vi "rsidr_core_global.vi"() -> ()   [LabVIEW 2020, in "Rohde&Schwarz RTx Oscilloscopes.lvlib"] (continued)
"Read Callback"="", "Write Callback"="", "Supported Models"="", "Instrument Options"="", "Flags"=0, "Help"="Defines the cursor measurement type.\n\nAvailable Repeated Capabilities:\nNone\n\nRemote-control command(s):\nCURSor<m>:FUNCtion"}, {"Level"=2, "Class Only"=FALSE, "Identifier"="RSRTX_ATTR_CURSOR_SOURCE", "Descriptive Name"="Cursor Source", "Data Type"=0, "Command"="CURS1:SOUR", "Access"=2, "Range Table"="rsrtx_rngWaveformParameter", "Read Callback"="", "Write Callback"="", "Supported Models"="", "Instrument Options"="", "Flags"=0, "Help"="Defines the source of the cursor measurement.\n\nAvailable Repeated Capabilities:\nNone\n\nRemote-control command(s):\nCURSor<m>:SOURce"}, {"Level"=2, "Class Only"=FALSE, "Identifier"="RSRTX_ATTR_CURSOR_SECOND_SOURCE", "Descriptive Name"="Cursor Second Source", "Data Type"=0, "Command"="CURS:SSO", "Access"=2, "Range Table"="rsrtx_rngWaveformParameter", "Read Callback"="", "Write Callback"="", "Supported Models"="", "Instrument Options"="", "Flags"=0, "Help"="Selects the second cursor source.\n\nAvailable Repeated Capabilities:\nNone\n\nRemote-control command(s):\nCURSor<m>:SSOURce"}, {"Level"=2, "Class Only"=FALSE, "Identifier"="RSRTX_ATTR_CURSOR_SECOND_SOURCE_ENABLE", "Descriptive Name"="Cursor Second Source Enable", "Data Type"=3, "Command"="CURS:USS", "Access"=2, "Range Table"="", "Read Callback"="", "Write Callback"="", "Supported Models"="", "Instrument Options"="", "Flags"=0, "Help"="Enables the second cursor source. To select the second source, use RSRTX_ATTR_CURSOR_SECOND_SOURCE. If enabled, the second cursor measures on the second source. Using a second source, you can measure differences between two waveforms with cursors. Both sources must be in the same domain (time domain or frequency domain).\n\nAvailable Repeated Capabilities:\nNone\n\nRemote-control command(s):\nCURSor<m>:USSOURce"}, {"Level"=2, "Class Only"=FALSE, "Identifier"="RSRTX_ATTR_CURSOR_TRACKING", "Descriptive Name"="Cursor Tracking", "Data Type"=3, "Command"="CURS1:TRAC", "Access"=2, "Range Table"="", "Read Callback"="", "Write Callback"="", "Supported Models"="", "Instrument Options"="", "Flags"=0, "Help"="If set to ON, the horizontal cursor lines follow the waveform.\n\nAvailable Repeated Capabilities:\nNone\n\nRemote-control command(s):\nCURSor<m>:TRACking[:STATe]"}, {"Level"=2, "Class Only"=FALSE, "Identifier"="RSRTX_ATTR_CURSOR_X_POSITION_COUPLING", "Descriptive Name"="Cursor X Position Coupling", "Data Type"=3, "Command"="CURS1:XCO", "Access"=2, "Range Table"="", "Read Callback"="", "Write Callback"="", "Supported Models"="", "Instrument Options"="", "Flags"=0, "Help"="Defines the positioning mode of the vertical cursor. \nON: Moving one cursor line moves the other cursor line too. The cursor lines always remain a fixed distance.\nOFF: Each cursor line is positioned independently.\n\nAvailable Repeated Capabilities:\nNone\n\nRemote-control command(s):\nCURSor<m>:XCOupling"}, {"Level"=2, "Class Only"=FALSE, "Identifier"="RSRTX_ATTR_CURSOR_Y_POSITION_COUPLING", "Descriptive Name"="Cursor Y Position Coupling", "Data Type"=3, "Command"="CURS:YCO", "Access"=2, "Range Table"="", "Read Callback"="", "Write Callback"="", "Supported Models"="", "Instrument Options"="", "Flags"=0, "Help"="Defines the positioning mode of the horizontal cursor. If the horizontal cursor lines track the waveform, the y-coupling is irrelevant.\nON: Moving one cursor line moves the other cursor line too. The cursor lines always remain a fixed distance.\nOFF: Each cursor line is positioned independently.\n\nAvailable Repeated Capabilities:\nNone\n\nRemote-control command(s):\nCURSor<m>:YCOupling"}, {"Level"=2, "Class Only"=FALSE, "Identifier"="RSRTX_ATTR_CURSOR_ADJUSTMENT", "Descriptive Name"="Cursor Adjustment", "Data Type"=3, "Command"="CURS1:TRAC:SCAL", "Access"=2, "Range Table"="", "Read Callback"="", "Write Callback"="", "Supported Models"="", "Instrument Options"="", "Flags"=0, "Help"="Enables the adjustment of cursor lines if the vertical or horizontal scales are changed.\n\nAvailable Repeated Capabilities:\nNone\n\nRemote-control command(s):\nCURSor<m>:TRACking:SCALe[:STATe]"}, {"Level"=2, "Class Only"=FALSE, "Identifier"="RSRTX_ATTR_CURSOR_X_RATIO_MEASUREMENT_UNIT", "Descriptive Name"="Cursor X Ratio Measurement Unit", "Data Type"=0, "Command"="CURS1:XRAT:UNIT", "Access"=2, "Range Table"="rsrtx_rngXRatioMeasurementUnit", "Read Callback"="", "Write Callback"="", "Supported Models"="", "Instrument Options"="", "Flags"=0, "Help"="Sets the unit for X Ratio measurements.\n\nAvailable Repeated Capabilities:\nNone\n\nRemote-control command(s):\nCURsor<m>:XRATio:UNIT"}, {"Level"=2, "Class Only"=FALSE, "Identifier"="RSRTX_ATTR_CURSOR_Y_RATIO_MEASUREMENT_UNIT", "Descriptive Name"="Cursor Y Ratio Measurement Unit", "Data Type"=0, "Command"="CURS1:YRAT:UNIT", "Access"=2, "Range Table"="rsrtx_rngYRatioMeasurementUnit", "Read Callback"="", "Write Callback"="", "Supported Models"="", "Instrument Options"="", "Flags"=0, "Help"="Sets the unit for Y Ratio measurements.\n\nAvailable Repeated Capabilities:\nNone\n\nRemote-control command(s):\nCURSor<m>:YRATio:UNIT"}, {"Level"=2, "Class Only"=FALSE, "Identifier"="RSRTX_ATTR_CURSOR_X_RATIO_MEASUREMENT", "Descriptive Name"="Cursor X Ratio Measurement", "Data Type"=1, "Command"="CURS1:XRAT?", "Access"=0, "Range Table"="", "Read Callback"="", "Write Callback"="", "Supported Models"="", "Instrument Options"="", "Flags"=0, "Help"="Returns the ratio of the x-values (e.g. a duty cycle) between the first and second cursors and the first and third cursors: (x2-x1)/(x3-x1).\n\nAvailable Repeated Capabilities:\nNone\n\nRemote-control command(s):\nCURSor<m>:XRATio[:VALue]?"}, {"Level"=2, "Class Only"=FALSE, "Identifier"="RSRTX_ATTR_CURSOR_Y_RATIO_MEASUREMENT", "Descriptive Name"="Cursor Y Ratio Measurement", "Data Type"=1, "Command"="CURS1:YRAT?", "Access"=0, "Range Table"="", "Read Callback"="", "Write Callback"="", "Supported Models"="", "Instrument Options"="", "Flags"=0, "Help"="Provides three cursors and measures the ratio of the y-values (e.g. overshooting) between the first and second cursors and the first and third cursors: (y2-y1)/(y3-y1).\n\nAvailable Repeated Capabilities:\nNone\n\nRemote-control command(s):\nCURSor<m>:YRATio[:VALue]?"}, {"Level"=2, "Class Only"=FALSE, "Identifier"="RSRTX_ATTR_CURSOR_DISTANCE_HORIZONTAL", "Descriptive Name"="Cursor Distance Horizontal", "Data Type"=1, "Command"="CURS1:XDEL?", "Access"=0, "Range Table"="", "Read Callback"="", "Write Callback"="", "Supported Models"="", "Instrument Options"="", "Flags"=0, "Help"="Queries the delta value (distance) of two horizontal cursors.\n\nAvailable Repeated Capabilities:\nNone\n\nRemote-control command(s):\nCURSor<m>:XDELta[:VALue]?"}, {"Level"=2, "Class Only"=FALSE, "Identifier"="RSRTX_ATTR_CURSOR_DISTANCE_VERTICAL", "Descriptive Name"="Cursor Distance Vertical", "Data Type"=1, "Command"="CURS1:YDEL?", "Access"=0, "Range Table"="", "Read Callback"="", "Write Callback"="", "Supported Models"="", "Instrument Options"="", "Flags"=0, "Help"="Queries the delta value (distance) of two vertical cursors.\n\nAvailable Repeated Capabilities:\nNone\n\nRemote-control command(s):\nCURSor<m>:YDELta[:VALue]?"}, {"Level"=2, "Class Only"=FALSE, "Identifier"="RSRTX_ATTR_CURSOR_INVERSE_DISTANCE", "Descriptive Name"="Cursor Inverse Distance", "Data Type"=1, "Command"="CURS1:XDEL:INV?", "Access"=0, "Range Table"="", "Read Callback"="", "Write Callback"="", "Supported Models"="", "Instrument Options"="", "Flags"=0, "Help"="Queries the inverse value of the delta value (distance) of the two vertical or horizontal cursors,\n\nAvailable Repeated Capabilities:\nNone\n\nRemote-control command(s):\nCURSor<m>:XDELta:INVerse?"}, {"Level"=2, "Class Only"=FALSE, "Identifier"="RSRTX_ATTR_CURSOR_VOLTAGE_INVERSE_DISTANCE_VERTICAL", "Descriptive Name"="Cursor Voltage Inverse Distance Vertical", "Data Type"=1, "Command"="CURS1:YDEL:SLOP?", "Access"=0, "Range Table"="", "Read Callback"="", "Write Callback"="", "Supported Models"="", "Instrument Options"="", "Flags"=1, "Help"="Returns the inverse value of the voltage difference - the reciprocal of the vertical distance of two horizontal cursor lines: 1/?V.\n\nAvailable Repeated Capabilities:\nNone\n\nRemote-control command(s):\nCURSor<m>:YDELta:SLOPe?"}, {"Level"=2, "Class Only"=FALSE, "Identifier"="RSRTX_ATTR_CURSOR_POSITION", "Descriptive Name"="Cursor Position", "Data Type"=1, "Command"="CURS1:RESult?", "Access"=0, "Range Table"="", "Read Callback"="", "Write Callback"="", "Supported Models"="", "Instrument Options"="", "Flags"=1, "Help"="Returns the cursor positions.\n\nAvailable Repeated Capabilities:\nNone\n\nRemote-control command(s):\nCURSor<m>:RESult?"}, {"Level"=2, "Class Only"=FALSE, "Identifier"="RSRTX_ATTR_CURSOR_AUTOSET", "Descriptive Name"="Cursor Autoset", "Data Type"=4, "Command"="CURS{Cursor}:SWAV", "Access"=1, "Range Table"="", "Read Callback"="", "Write Callback"="", "Supported Models"="", "Instrument Options"="", "Flags"=1, "Help"="Sets the cursor lines to typical points of the waveform depending on the selected measurement type.\n\nAvailable Repeated Capabilities:\nCursor: Cur1, Cur2, Cur3\r\n\nRemote-control command(s):\nCURSor<m>:SWAVe"}, {"Level"=2, "Class Only"=FALSE, "Identifier"="RSRTX_ATTR_CURSOR_RESET", "Descriptive Name"="Cursor Reset", "Data Type"=4, "Command"="CURS{Cursor}:SSCR", "Access"=1, "Range Table"="", "Read Callback"="", "Write Callback"="", "Supported Models"="", "Instrument Options"="", "Flags"=0, "Help"="Resets the cursors to their initial positions.\n\nAvailable Repeated Capabilities:\nCursor: Cur1, Cur2, Cur3\r\n\nRemote-control command(s):\nCURSor<m>:SSCReen"}, {"Level"=2, "Class Only"=FALSE, "Identifier"="RSRTX_ATTR_CURSOR_PEAK_NEXT", "Descriptive Name"="Cursor Peak Next", "Data Type"=4, "Command"="CURS{Cursor}:SNP", "Access"=1, "Range Table"="", "Read Callback"="", "Write Callback"="", "Supported Models"="", "Instrument Options"="", "Flags"=0, "Help"="Sets cursor to the next peak.\n\nAvailable Repeated Capabilities:\nCursor: Cur1, Cur2, Cur3\r\n\nRemote-control command(s):\nCURSor<m>:SNPeak"}, {"Level"=2, "Class Only"=FALSE, "Identifier"="RSRTX_ATTR_CURSOR_PEAK_PREVIOUS", "Descriptive Name"="Cursor Peak Previous", "Data Type"=4, "Command"="CURS{Cursor}:SPP", "Access"=1, "Range Table"="", "Read Callback"="", "Write Callback"="", "Supported Models"="", "Instrument Options"="", "Flags"=0, "Help"="Sets cursor to the previous peak.\n\nAvailable Repeated Capabilities:\nCursor: Cur1, Cur2, Cur3\r\n\nRemote-control command(s):\nCURSor<m>:SPPeak"}, {"Level"=2, "Class Only"=FALSE, "Identifier"="RSRTX_ATTR_CURSOR_X1_POSITION", "Descriptive Name"="Cursor X1 Position", "Data Type"=1, "Command"="CURS1:X1P", "Access"=2, "Range Table"="rsrtx_rngCursorXPosition", "Read Callback"="", "Write Callback"="", "Supported Models"="", "Instrument Options"="", "Flags"=0, "Help"="Defines the vertical position of first cursor or cursor line.\n\nAvailable Repeated Capabilities:\nNone\n\nRemote-control command(s):\nCURSor<m>:X1Position"}, {"Level"=2, "Class Only"=FALSE, "Identifier"="RSRTX_ATTR_CURSOR_X2_POSITION", "Descriptive Name"="Cursor X2 Position", "Data Type"=1, "Command"="CURS1:X2P", "Access"=2, "Range Table"="rsrtx_rngCursorXPosition", "Read Callback"="", "Write Callback"="", "Supported Models"="", "Instrument Options"="", "Flags"=0, "Help"="Defines the vertical position of second cursor or cursor line.\n\nAvailable Repeated Capabilities:\nNone\n\nRemote-control command(s):\nCURSor<m>:X2Position"}, {"Level"=2, "Class Only"=FALSE, "Identifier"="RSRTX_ATTR_CURSOR_X3_POSITION", "Descriptive Name"="Cursor X3 Position", "Data Type"=1, "Command"="CURS1:X3P", "Access"=2, "Range Table"="rsrtx_rngCursorXPosition", "Read Callback"="", "Write Callback"="", "Supported Models"="", "Instrument Options"="", "Flags"=0, "Help"="Defines the vertical position of third cursor or cursor line.\n\nAvailable Repeated Capabilities:\nNone\n\nRemote-control command(s):\nCURSor<m>:X3Position"}, {"Level"=2, "Class Only"=FALSE, "Identifier"="RSRTX_ATTR_CURSOR_Y1_POSITION", "Descriptive Name"="Cursor Y1 Position", "Data Type"=1, "Command"="CURS1:Y1P", "Access"=2, "Range Table"="rsrtx_rngCursorYPosition", "Read Callback"="", "Write Callback"="", "Supported Models"="", "Instrument Options"="", "Flags"=0, "Help"="Defines the horizontal position of first cursor or cursor line.\n\nAvailable Repeated Capabilities:\nNone\n\nRemote-control command(s):\nCURSor<m>:Y1Position"}, {"Level"=2, "Class Only"=FALSE, "Identifier"="RSRTX_ATTR_CURSOR_Y2_POSITION", "Descriptive Name"="Cursor Y2 Position", "Data Type"=1, "Command"="CURS1:Y2P", "Access"=2, "Range Table"="rsrtx_rngCursorYPosition", "Read Callback"="", "Write Callback"="", "Supported Models"="", "Instrument Options"="", "Flags"=0, "Help"="Defines the horizontal position of second cursor or cursor line.\n\nAvailable Repeated Capabilities:\nNone\n\nRemote-control command(s):\nCURSor<m>:Y2Position"}, {"Level"=2, "Class Only"=FALSE, "Identifier"="RSRTX_ATTR_CURSOR_Y3_POSITION", "Descriptive Name"="Cursor Y3 Position", "Data Type"=1, "Command"="CURS1:Y3P", "Access"=2, "Range Table"="rsrtx_rngCursorYPosition", "Read Callback"="", "Write Callback"="", "Supported Models"="", "Instrument Options"="", "Flags"=0, "Help"="Defines the horizontal position of third cursor or cursor line.\n\nAvailable Repeated Capabilities:\nNone\n\nRemote-control command(s):\nCURSor<m>:Y3Position"}, {"Level"=2, "Class Only"=TRUE, "Identifier"="", "Descriptive Name"="Cursor Line", "Data Type"=0, "Command"="", "Access"=0, "Range Table"="", "Read Callback"="", "Write Callback"="", "Supported Models"="", "Instrument Options"="", "Flags"=0, "Help"="Class for CursorLine repcap."}, {"Level"=3, "Class Only"=FALSE, "Identifier"="RSRTX_ATTR_CURSOR_LINE_NEXT_PEAK", "Descriptive Name"="Cursor Line Next Peak", "Data Type"=4, "Command"="CURS{Cursor}:SNP{CursorLine}", "Access"=1, "Range Table"="", "Read Callback"="", "Write Callback"="", "Supported Models"="", "Instrument Options"="", "Flags"=0, "Help"="Set the cursor line to the next peak, respectively. Only available for FFT waveforms.\n\nAvailable Repeated Capabilities:\nCursor: Cur1, Cur2, Cur3\r\nCursorLine: CursorLine1, CursorLine2\r\n\nRemote-control command(s):\nCURSor<m>:SNPeak<n>"}, {"Level"=3, "Class Only"=FALSE, "Identifier"="RSRTX_ATTR_CURSOR_LINE_PREVIOUS_PEAK", "Descriptive Name"="Cursor Line Previous Peak", "Data Type"=4, "Command"="CURS{Cursor}:SPP{CursorLine}", "Access"=1, "Range Table"="", "Read Callback"="", "Write Callback"="", "Supported Models"="", "Instrument Options"="", "Flags"=0, "Help"="Set the cursor line to the previous peak, respectively. Only available for FFT waveforms.\n\nAvailable Repeated Capabilities:\nCursor: Cur1, Cur2, Cur3\r\nCursorLine: CursorLine1, CursorLine2\r\n\nRemote-control command(s):\nCURSor<m>:SPPeak<n>"}, {"Level"=1, "Class Only"=TRUE, "Identifier"="", "Descriptive Name"="Measurements", "Data Type"=0, "Command"="", "Access"=0, "Range Table"="", "Read Callback"="", "Write Callback"="", "Supported Models"="", "Instrument Options"="", "Flags"=0, "Help"="Configures scope measurements and queries results."}, {"Level"=2, "Class Only"=FALSE, "Identifier"="RSRTX_ATTR_MEAS_RELATIVE_MODE", "Descriptive Name"="Measurement Relative Mode", "Data Type"=0, "Command"="REFL:REL:MODE", "Access"=2, "Range Table"="rsrtx_rngRelativeMode", "Read Callback"="", "Write Callback"="", "Supported Models"="", "Instrument Options"="", "Flags"=0, "Help"="Sets the lower and upper reference levels for rise and fall time mesurements (cursor and automatic mesurements) as well as the middle reference level for phase and delay measurements. The levels are defined as percentages of the high signal level. The setting is valid for all measurement places.\n\nAvailable Repeated Capabilities:\nNone\n\nRemote-control command(s):\nREFLevel:RELative:MODE"}, {"Level"=2, "Class Only"=FALSE, "Identifier"="RSRTX_ATTR_MEAS_RELATIVE_LOWER_LEVEL", "Descriptive Name"="Measurement Relative Lower Level", "Data Type"=1, "Command"="REFL:REL:LOW", "Access"=2, "Range Table"="rsrtx_rngRelLevel", "Read Callback"="", "Write Callback"="", "Supported Models"="", "Instrument Options"="", "Flags"=0, "Help"="Set the lower reference level for rise and fall time mesurements.\n\nAvailable Repeated Capabilities:\nNone\n\nRemote-control command(s):\nREFLevel:RELative:LOWer"}, {"Level"=2, "Class Only"=FALSE, "Identifier"="RSRTX_ATTR_MEAS_RELATIVE_UPPER_LEVEL", "Descriptive Name"="Measurement Relative Upper Level", "Data Type"=1, "Command"="REFL:REL:UPP", "Access"=2, "Range Table"="rsrtx_rngRelLevel", "Read Callback"="", "Write Callback"="", "Supported Models"="", "Instrument Options"="", "Flags"=0, "Help"="Set the upper reference level for rise and fall time mesurements.\n\nAvailable Repeated Capabilities:\nNone\n\nRemote-control command(s):\nREFLevel:RELative:UPPer"}, {"Level"=2, "Class Only"=FALSE, "Identifier"="RSRTX_ATTR_MEAS_RELATIVE_MIDDLE_LEVEL", "Descriptive Name"="Measurement Relative Middle Level", "Data Type"=1, "Command"="REFL:REL:MIDD", "Access"=2, "Range Table"="rsrtx_rngRelLevel", "Read Callback"="", "Write Callback"="", "Supported Models"="", "Instrument Options"="", "Flags"=0, "Help"="Set the middle reference level used for phase and delay measurements.\n\nAvailable Repeated Capabilities:\nNone\n\nRemote-control command(s):\nREFLevel:RELative:MIDDle"}, {"Level"=2, "Class Only"=TRUE, "Identifier"="", "Descriptive Name"="Main Measurements", "Data Type"=0, "Command"="", "Access"=0, "Range Table"="", "Read Callback"="", "Write Callback"="", "Supported Models"="", "Instrument Options"="", "Flags"=0, "Help"="Configures scope measurements and queries results."}, {"Level"=3, "Class Only"=FALSE, "Identifier"="RSRTX_ATTR_MAIN_MEASUREMENT_RESULT_FREQUENCY", "Descriptive Name"="Main Measurement Result Frequency", "Data Type"=1, "Command"="MEAS{Measurement}:RES? FREQ", "Access"=0, "Range Table"="", "Read Callback"="", "Write Callback"="", "Supported Models"="", "Instrument Options"="", "Flags"=0, "Help"="Returns the result of the frequency measurement type.\n\nAvailable Repeated Capabilities:\nMeasurement: M1, M2, M3, M4, M5, M6, M7, M8\r\n\nRemote-control command(s):\nMEASurement<m>:RESult[:ACTual]?"}, {"Level"=3, "Class Only"=FALSE, "Identifier"="RSRTX_ATTR_MAIN_MEASUREMENT_RESULT_PERIOD", "Descriptive Name"="Main Measurement Result Period", "Data Type"=1, "Command"="MEAS{Measurement}:RES? PER", "Access"=0, "Range Table"="", "Read Callback"="", "Write Callback"="", "Supported Models"="", "Instrument Options"="", "Flags"=0, "Help"="Returns the result of the period measurement type.\n\nAvailable Repeated Capabilities:\nMeasurement: M1, M2, M3, M4, M5, M6, M7, M8\r\n\nRemote-control command(s):\nMEASurement<m>:RESult[:ACTual]?"}, {"Level"=3, "Class Only"=FALSE, "Identifier"="RSRTX_ATTR_MAIN_MEASUREMENT_RESULT_PEAK", "Descriptive Name"="Main Measurement Result Peak", "Data Type"=1, "Command"="MEAS{Measurement}:RES? PEAK", "Access"=0, "Range Table"="", "Read Callback"="", "Write Callback"="", "Supported Models"="", "Instrument Options"="", "Flags"=0, "Help"="Returns the result of the peak measurement type.\n\nAvailable Repeated Capabilities:\nMeasurement: M1, M2, M3, M4, M5, M6, M7, M8\r\n\nRemote-control command(s):\nMEASurement<m>:RESult[:ACTual]?"}, {"Level"=3, "Class Only"=FALSE, "Identifier"="RSRTX_ATTR_MAIN_MEASUREMENT_RESULT_MAXIMUM_PEAK", "Descriptive Name"="Main Measurement Result Maximum Peak", "Data Type"=1, "Command"="MEAS{Measurement}:RES? UPE", "Access"=0, "Range Table"="", "Read Callback"="", "Write Callback"="", "Supported Models"="", "Instrument Options"="", "Flags"=0, "Help"="Returns the result of the maximum peak measurement type.\n\nAvailable Repeated Capabilities:\nMeasurement: M1, M2, M3, M4, M5, M6, M7, M8\r\n\nRemote-control command(s):\nMEASurement<m>:RESult[:ACTual]?"}, {"Level"=3, "Class Only"=FALSE, "Identifier"="RSRTX_ATTR_MAIN_MEASUREMENT_RESULT_MINIMUM_PEAK", "Descriptive Name"="Main Measurement Result Minimum Peak", "Data Type"=1, "Command"="MEAS{Measurement}:RES? LPE", "Access"=0, "Range Table"="", "Read Callback"="", "Write Callback"="", "Supported Models"="", "Instrument Options"="", "Flags"=0, "Help"="Returns the result of the minimum peak measurement type.\n\nAvailable Repeated Capabilities:\nMeasurement: M1, M2, M3, M4, M5, M6, M7, M8\r\n\nRemote-control command(s):\nMEASurement<m>:RESult[:ACTual]?"}, {"Level"=3, "Class Only"=FALSE, "Identifier"="RSRTX_ATTR_MAIN_MEASUREMENT_RESULT_POSITIVE_PULSES", "Descriptive Name"="Main Measurement Result Positive Pulses", "Data Type"=1, "Command"="MEAS{Measurement}:RES? PPC", "Access"=0, "Range Table"="", "Read Callback"="", "Write Callback"="", "Supported Models"="", "Instrument Options"="", "Flags"=0, "Help"="Returns the result of the positive pulses measurement type.\n\nAvailable Repeated Capabilities:\nMeasurement: M1, M2, M3, M4, M5, M6, M7, M8\r\n\nRemote-control command(s):\nMEASurement<m>:RESult[:ACTual]?"}, {"Level"=3, "Class Only"=FALSE, "Identifier"="RSRTX_ATTR_MAIN_MEASUREMENT_RESULT_NEGATIVE_PULSES", "Descriptive Name"="Main Measurement Result Negative Pulses", "Data Type"=1, "Command"="MEAS{Measurement}:RES? NPC", "Access"=0, "Range Table"="", "Read Callback"="", "Write Callback"="", "Supported Models"="", "Instrument Options"="", "Flags"=0, "Help"="Returns the result of the negative pulses measurement type.\n\nAvailable Repeated Capabilities:\nMeasurement: M1, M2, M3, M4, M5, M6, M7, M8\r\n\nRemote-control command(s):\nMEASurement<m>:RESult[:ACTual]?"}, {"Level"=3, "Class Only"=FALSE, "Identifier"="RSRTX_ATTR_MAIN_MEASUREMENT_RESULT_RISING_EDGES", "Descriptive Name"="Main Measurement Result Rising Edges", "Data Type"=1, "Command"="MEAS{Measurement}:RES? REC", "Access"=0, "Range Table"="", "Read Callback"="", "Write Callback"="", "Supported Models"="", "Instrument Options"="", "Flags"=0, "Help"="Returns the result of the rising edges measurement type.\n\nAvailable Repeated Capabilities:\nMeasurement: M1, M2, M3, M4, M5, M6, M7, M8\r\n\nRemote-control command(s):\nMEASurement<m>:RESult[:ACTual]?"}, {"Level"=3, "Class Only"=FALSE, "Identifier"="RSRTX_ATTR_MAIN_MEASUREMENT_RESULT_FALLING_EDGES", "Descriptive Name"="Main Measurement Result Falling Edges", "Data Type"=1, "Command"="MEAS{Measurement}:RES? FEC", "Access"=0, "Range Table"="", "Read Callback"="", "Write Callback"="", "Supported Models"="", "Instrument Options"="", "Flags"=0, "Help"="Returns the result of the falling edges measurement type.\n\nAvailable Repeated Capabilities:\nMeasurement: M1, M2, M3, M4, M5, M6, M7, M8\r\n\nRemote-control command(s):\nMEASurement<m>:RESult[:ACTual]?"}, {"Level"=3, "Class Only"=FALSE, "Identifier"="RSRTX_ATTR_MAIN_MEASUREMENT_RESULT_HIGH_LEVEL", "Descriptive Name"="Main Measurement Result High Level", "Data Type"=1, "Command"="MEAS{Measurement}:RES? HIGH", "Access"=0, "Range Table"="", "Read Callback"="", "Write Callback"="", "Supported Models"="", "Instrument Options"="", "Flags"=0, "Help"="Returns the result of the high level measurement type.\n\nAvailable Repeated Capabilities:\nMeasurement: M1, M2, M3, M4, M5, M6, M7, M8\r\n\nRemote-control command(s):\nMEASurement<m>:RESult[:ACTual]?"}, {"Level"=3, "Class Only"=FALSE, "Identifier"="RSRTX_ATTR_MAIN_MEASUREMENT_RESULT_LOW_LEVEL", "Descriptive Name"="Main Measurement Result Low Level", "Data Type"=1, "Command"="MEAS{Measurement}:RES? LOW", "Access"=0, "Range Table"="", "Read Callback"="", "Write Callback"="", "Supported Models"="", "Instrument Options"="", "Flags"=0, "Help"="Returns the result of the low level measurement type.\n\nAvailable Repeated Capabilities:\nMeasurement: M1, M2, M3, M4, M5, M6, M7, M8\r\n\nRemote-control command(s):\nMEASurement<m>:RESult[:ACTual]?"}, {"Level"=3, "Class Only"=FALSE, "Identifier"="RSRTX_ATTR_MAIN_MEASUREMENT_RESULT_AMPLITUDE", "Descriptive Name"="Main Measurement Result Amplitude", "Data Type"=1, "Command"="MEAS{Measurement}:RES? AMPL", "Access"=0, "Range Table"="", "Read Callback"="", "Write Callback"="", "Supported Models"="", "Instrument Options"="", "Flags"=0, "Help"="Returns the result of the amplitude measurement type.\n\nAvailable Repeated Capabilities:\nMeasurement: M1, M2, M3, M4, M5, M6, M7, M8\r\n\nRemote-control command(s):\nMEASurement<m>:RESult[:ACTual]?"}, {"Level"=3, "Class Only"=FALSE, "Identifier"="RSRTX_ATTR_MAIN_MEASUREMENT_RESULT_MEAN", "Descriptive Name"="Main Measurement Result Mean", "Data Type"=1, "Command"="MEAS{Measurement}:RES? MEAN", "Access"=0, "Range Table"="", "Read Callback"="", "Write Callback"="", "Supported Models"="", "Instrument Options"="", "Flags"=0, "Help"="Returns the result of the mean measurement type.\n\nAvailable Repeated Capabilities:\nMeasurement: M1, M2, M3, M4, M5, M6, M7, M8\r\n\nRemote-control command(s):\nMEASurement<m>:RESult[:ACTual]?"}, {"Level"=3, "Class Only"=FALSE, "Identifier"="RSRTX_ATTR_MAIN_MEASUREMENT_RESULT_RMS", "Descriptive Name"="Main Measurement Result RMS", "Data Type"=1, "Command"="MEAS{Measurement}:RES? RMS", "Access"=0, "Range Table"="", "Read Callback"="", "Write Callback"="", "Supported Models"="", "Instrument Options"="", "Flags"=0, "Help"="Returns the result of the RMS measurement type.\n\nAvailable Repeated Capabilities:\nMeasurement: M1, M2, M3, M4, M5, M6, M7, M8\r\n\nRemote-control command(s):\nMEASurement<m>:RESult[:ACTual]?"}, {"Level"=3, "Class Only"=FALSE, "Identifier"="RSRTX_ATTR_MAIN_MEASUREMENT_RESULT_RISE_TIME", "Descriptive Name"="Main Measurement Result Rise Time", "Data Type"=1, "Command"="MEAS{Measurement}:RES? RTIM", "Access"=0, "Range Table"="", "Read Callback"="", "Write Callback"="", "Supported Models"="", "Instrument Options"="", "Flags"=0, "Help"="Returns the result of the rise time measurement type.\n\nAvailable Repeated Capabilities:\nMeasurement: M1, M2, M3, M4, M5, M6, M7, M8\r\n\nRemote-control command(s):\nMEASurement<m>:RESult[:ACTual]?"}, {"Level"=3, "Class Only"=FALSE, "Identifier"="RSRTX_ATTR_MAIN_MEASUREMENT_RESULT_FALLING_TIME", "Descriptive Name"="Main Measurement Result Falling Time", "Data Type"=1, "Command"="MEAS{Measurement}:RES? FTIM", "Access"=0, "Range Table"="", "Read Callback"="", "Write Callback"="", "Supported Models"="", "Instrument Options"="", "Flags"=0, "Help"="Returns the result of the falling time measurement type.\n\nAvailable Repeated Capabilities:\nMeasurement: M1, M2, M3, M4, M5, M6, M7, M8\r\n\nRemote-control command(s):\nMEASurement<m>:RESult[:ACTual]?"}, {"Level"=3, "Class Only"=FALSE, "Identifier"="RSRTX_ATTR_MAIN_MEASUREMENT_RESULT_POSITIVE_CYCLE", "Descriptive Name"="Main Measurement Result Positive Cycle", "Data Type"=1, "Command"="MEAS{Measurement}:RES? PDCY", "Access"=0, "Range Table"="", "Read Callback"="", "Write Callback"="", "Supported Models"="", "Instrument Options"="", "Flags"=0, "Help"="Returns the result of the positive cycle measurement type.\n\nAvailable Repeated Capabilities:\nMeasurement: M1, M2, M3, M4, M5, M6, M7, M8\r\n\nRemote-control command(s):\nMEASurement<m>:RESult[:ACTual]?"}, {"Level"=3, "Class Only"=FALSE, "Identifier"="RSRTX_ATTR_MAIN_MEASUREMENT_RESULT_NEGATIVE_CYCLE", "Descriptive Name"="Main Measurement Result Negative Cycle", "Data Type"=1, "Command"="MEAS{Measurement}:RES? NDCY", "Access"=0, "Range Table"="", "Read Callback"="", "Write Callback"="", "Supported Models"="", "Instrument Options"="", "Flags"=0, "Help"="Returns the result of the negative cycle measurement type.\n\nAvailable Repeated Capabilities:\nMeasurement: M1, M2, M3, M4, M5, M6, M7, M8\r\n\nRemote-control command(s):\nMEASurement<m>:RESult[:ACTual]?"}, {"Level"=3, "Class Only"=FALSE, "Identifier"="RSRTX_ATTR_MAIN_MEASUREMENT_RESULT_WIDTH_POSITIVE_PULSE", "Descriptive Name"="Main Measurement Result Width Positive Pulse", "Data Type"=1, "Command"="MEAS{Measurement}:RES? PPW", "Access"=0, "Range Table"="", "Read Callback"="", "Write Callback"="", "Supported Models"="", "Instrument Options"="", "Flags"=0, "Help"="Returns the result of the width of the positive pulse measurement type.\n\nAvailable Repeated Capabilities:\nMeasurement: M1, M2, M3, M4, M5, M6, M7, M8\r\n\nRemote-control command(s):\nMEASurement<m>:RESult[:ACTual]?"}, {"Level"=3, "Class Only"=FALSE, "Identifier"="RSRTX_ATTR_MAIN_MEASUREMENT_RESULT_WIDTH_NEGATIVE_PULSE", "Descriptive Name"="Main Measurement Result Width Negative Pulse", "Data Type"=1, "Command"="MEAS{Measurement}:RES? NPW", "Access"=0, "Range Table"="", "Read Callback"="", "Write Callback"="", "Supported Models"="", "Instrument Options"="", "Flags"=0, "Help"="Returns the result of the width of the negative pulse measurement type.\n\nAvailable Repeated Capabilities:\nMeasurement: M1, M2, M3, M4, M5, M6, M7, M8\r\n\nRemote-control command(s):\nMEASurement<m>:RESult[:ACTual]?"}, {"Level"=3, "Class Only"=FALSE, "Identifier"="RSRTX_ATTR_MAIN_MEASUREMENT_RESULT_MEAN_VALUE", "Descriptive Name"="Main Measurement Result Mean Value", "Data Type"=1, "Command"="MEAS{Measurement}:RES? CYCM", "Access"=0, "Range Table"="", "Read Callback"="", "Write Callback"="", "Supported Models"="", "Instrument Options"="", "Flags"=0, "Help"="Returns the result of the width of the mean value measurement type.\n\nAvailable Repeated Capabilities:\nMeasurement: M1, M2, M3, M4, M5, M6, M7, M8\r\n\nRemote-control command(s):\nMEASurement<m>:RESult[:ACTual]?"}, {"Level"=3, "Class Only"=FALSE, "Identifier"="RSRTX_ATTR_MAIN_MEASUREMENT_RESULT_RMS_VALUE", "Descriptive Name"="Main Measurement Result RMS Value", "Data Type"=1, "Command"="MEAS{Measurement}:RES? CYCR", "Access"=0, "Range Table"="", "Read Callback"="", "Write Callback"="", "Supported Models"="", "Instrument Options"="", "Flags"=0, "Help"="Returns the result of the width of the RMS value measurement type.\n\nAvailable Repeated Capabilities:\nMeasurement: M1, M2, M3, M4, M5, M6, M7, M8\r\n\nRemote-control command(s):\nMEASurement<m>:RESult[:ACTual]?"}, {"Level"=3, "Class Only"=FALSE, "Identifier"="RSRTX_ATTR_MAIN_MEASUREMENT_RESULT_STANDARD_DEVIATIONS", "Descriptive Name"="Main Measurement Result Standard Deviations", "Data Type"=1, "Command"="MEAS{Measurement}:RES? STDD", "Access"=0, "Range Table"="", "Read Callback"="", "Write Callback"="", "Supported Models"="", "Instrument Options"="", "Flags"=0, "Help"="Returns the result of the width of the standard deviation measurement type.\n\nAvailable Repeated Capabilities:\nMeasurement: M1, M2, M3, M4, M5, M6, M7, M8\r\n\nRemote-control command(s):\nMEASurement<m>:RESult[:ACTual]?"}, {"Level"=3, "Class Only"=FALSE, "Identifier"="RSRTX_ATTR_MAIN_MEASUREMENT_RESULT_STANDARD_DEVIATION_VALUE", "Descriptive Name"="Main Measurement Result Standard Deviation Value", "Data Type"=1, "Command"="MEAS{Measurement}:RES? CYCS", "Access"=0, "Range Table"="", "Read Callback"="", "Write Callback"="", "Supported Models"="", "Instrument Options"="", "Flags"=0, "Help"="Returns the result of the width of the standard deviation value measurement type.\n\nAvailable Repeated Capabilities:\nMeasurement: M1, M2, M3, M4, M5, M6, M7, M8\r\n\nRemote-control command(s):\nMEASurement<m>:RESult[:ACTual]?"}, {"Level"=3, "Class Only"=FALSE, "Identifier"="RSRTX_ATTR_MAIN_MEASUREMENT_RESULT_DELAY", "Descriptive Name"="Main Measurement Result Delay", "Data Type"=1, "Command"="MEAS{Measurement}:RES? DEL", "Access"=0, "Range Table"="", "Read Callback"="", "Write Callback"="", "Supported Models"="", "Instrument Options"="", "Flags"=0, "Help"="Returns the result of the width of the delay measurement type.\n\nAvailable Repeated Capabilities:\nMeasurement: M1, M2, M3, M4, M5, M6, M7, M8\r\n\nRemote-control command(s):\nMEASurement<m>:RESult[:ACTual]?"}, {"Level"=3, "Class Only"=FALSE, "Identifier"="RSRTX_ATTR_MAIN_MEASUREMENT_RESULT_PHASE", "Descriptive Name"="Main Measurement Result Phase", "Data Type"=1, "Command"="MEAS{Measurement}:RES? PHAS", "Access"=0, "Range Table"="", "Read Callback"="", "Write Callback"="", "Supported Models"="", "Instrument Options"="", "Flags"=0, "Help"="Returns the result of the width of the phase measurement type.\n\nAvailable Repeated Capabilities:\nMeasurement: M1, M2, M3, M4, M5, M6, M7, M8\r\n\nRemote-control command(s):\nMEASurement<m>:RESult[:ACTual]?"}, {"Level"=3, "Class Only"=FALSE, "Identifier"="RSRTX_ATTR_MAIN_MEASUREMENT_RESULT_BURST_WIDTH", "Descriptive Name"="Main Measurement Result Burst Width", "Data Type"=1, "Command"="MEAS{Measurement}:RES? BWID", "Access"=0, "Range Table"="", "Read Callback"="", "Write Callback"="", "Supported Models"="", "Instrument Options"="", "Flags"=0, "Help"="Returns the result of the width of the burst width measurement type.\n\nAvailable Repeated Capabilities:\nMeasurement: M1, M2, M3, M4, M5, M6, M7, M8\r\n\nRemote-control command(s):\nMEASurement<m>:RESult[:ACTual]?"}, {"Level"=3, "Class Only"=FALSE, "Identifier"="RSRTX_ATTR_MAIN_MEASUREMENT_RESULT_POSITIVE_OVERSHOOT", "Descriptive Name"="Main Measurement Result Positive Overshoot", "Data Type"=1, "Command"="MEAS{Measurement}:RES? POV", "Access"=0, "Range Table"="", "Read Callback"="", "Write Callback"="", "Supported Models"="", "Instrument Options"="", "Flags"=0, "Help"="Returns the result of the width of the positive overshoot measurement type.\n\nAvailable Repeated Capabilities:\nMeasurement: M1, M2, M3, M4, M5, M6, M7, M8\r\n\nRemote-control command(s):\nMEASurement<m>:RESult[:ACTual]?"}, {"Level"=3, "Class Only"=FALSE, "Identifier"="RSRTX_ATTR_MAIN_MEASUREMENT_RESULT_NEGATIVE_OVERSHOOT", "Descriptive Name"="Main Measurement Result Negative Overshoot", "Data Type"=1, "Command"="MEAS{Measurement}:RES? NOV", "Access"=0, "Range Table"="", "Read Callback"="", "Write Callback"="", "Supported Models"="", "Instrument Options"="", "Flags"=0, "Help"="Returns the result of the width of the negative overshoot measurement type.\n\nAvailable Repeated Capabilities:\nMeasurement: M1, M2, M3, M4, M5, M6, M7, M8\r\n\nRemote-control command(s):\nMEASurement<m>:RESult[:ACTual]?"}, {"Level"=3, "Class Only"=FALSE, "Identifier"="RSRTX_ATTR_MAIN_MEASUREMENT_RESULT_AVERAGE_VALUE", "Descriptive Name"="Main Measurement Result Average Value", "Data Type"=1, "Command"="MEAS{Measurement}:RES:AVG?", "Access"=0, "Range Table"="", "Read Callback"="", "Write Callback"="", "Supported Models"="", "Instrument Options"="", "Flags"=0, "Help"="Returns the result of the Average Value measurement type.\n\nAvailable Repeated Capabilities:\nMeasurement: M1, M2, M3, M4, M5, M6, M7, M8\r\n\nRemote-control command(s):\nMEASurement<m>:RESult:AVG?"}, {"Level"=3, "Class Only"=FALSE, "Identifier"="RSRTX_ATTR_MAIN_MEASUREMENT_RESULT_STANDARD_DEVIATION", "Descriptive Name"="Main Measurement Result Standard Deviation", "Data Type"=1, "Command"="MEAS{Measurement}:RES:STDD?", "Access"=0, "Range Table"="", "Read Callback"="", "Write Callback"="", "Supported Models"="", "Instrument Options"="", "Flags"=0, "Help"="Returns the result of the Standard Deviation measurement type.\n\nAvailable Repeated Capabilities:\nMeasurement: M1, M2, M3, M4, M5, M6, M7, M8\r\n\nRemote-control command(s):\nMEASurement<m>:RESult:STDDev?"}, {"Level"=3, "Class Only"=FALSE, "Identifier"="RSRTX_ATTR_MAIN_MEASUREMENT_RESULT_NEGATIVE_PEAK", "Descriptive Name"="Main Measurement Result Negative Peak", "Data Type"=1, "Command"="MEAS{Measurement}:RES:NPE?", "Access"=0, "Range Table"="", "Read Callback"="", "Write Callback"="", "Supported Models"="", "Instrument Options"="", "Flags"=0, "Help"="Returns the result of the Negative Peak measurement type.\n\nAvailable Repeated Capabilities:\nMeasurement: M1, M2, M3, M4, M5, M6, M7, M8\r\n\nRemote-control command(s):\nMEASurement<m>:RESult:NPEak?"}, {"Level"=3, "Class Only"=FALSE, "Identifier"="RSRTX_ATTR_MAIN_MEASUREMENT_RESULT_POSITIVE_PEAK", "Descriptive Name"="Main Measurement Result Positive Peak", "Data Type"=1, "Command"="MEAS{Measurement}:RES:PPE?", "Access"=0, "Range Table"="", "Read Callback"="", "Write Callback"="", "Supported Models"="", "Instrument Options"="", "Flags"=0, "Help"="Returns the result of the Positive Peak measurement type.\n\nAvailable Repeated Capabilities:\nMeasurement: M1, M2, M3, M4, M5, M6, M7, M8\r\n\nRemote-control command(s):\nMEASurement<m>:RESult:PPEak?"}, {"Level"=3, "Class Only"=FALSE, "Identifier"="RSRTX_ATTR_MAIN_MEASUREMENT_RESULT_WAVEFORM_COUNT", "Descriptive Name"="Main Measurement Result Waveform Count", "Data Type"=0, "Command"="MEAS{Measurement}:RES:WFMC?", "Access"=0, "Range Table"="", "Read Callback"="", "Write Callback"="", "Supported Models"="", "Instrument Options"="", "Flags"=0, "Help"="Returns the result of the Waveform Count measurement type.\n\nAvailable Repeated Capabilities:\nMeasurement: M1, M2, M3, M4, M5, M6, M7, M8\r\n\nRemote-control command(s):\nMEASurement<m>:RESult:WFMCount?"}, {"Level"=3, "Class Only"=FALSE, "Identifier"="RSRTX_ATTR_AMPT_MAIN_MEASUREMENT", "Descriptive Name"="Amplitude Time Main Measurement", "Data Type"=0, "Command"="MEAS{Measurement}:MAIN", "Access"=2, "Range Table"="rsrtx_rngAmplitudeTimeMeasurementType", "Read Callback"="", "Write Callback"="", "Supported Models"="", "Instrument Options"="", "Flags"=0, "Help"="Defines or queries the main measurement. This measurement is the one referred to if the measurement waveform is used as a source for math calculations. The main measurement type must belong to the same category as the other types assigned to the same measurement waveform, if there are any.\n\nAvailable Repeated Capabilities:\nMeasurement: M1, M2, M3, M4, M5, M6, M7, M8\r\n\nRemote-control command(s):\nMEASurement<m>:MAIN"}, {"Level"=3, "Class Only"=FALSE, "Identifier"="RSRTX_ATTR_MEASUREMENT_DELAY_MARKER_VISIBLE", "Descriptive Name"="Measurement Delay Marker Visible", "Data Type"=3, "Command"="MEAS{Measurement}:DEL:MARK", "Access"=2, "Range Table"="", "Read Callback"="", "Write Callback"="", "Supported Models"="", "Instrument Options"="", "Flags"=0, "Help"="If ON, the markers show the edge, the measured point on the edge, and the direction in which the edge is detected.\n\nAvailable Repeated Capabilities:\nMeasurement: M1, M2, M3, M4, M5, M6, M7, M8\r\n\nRemote-control command(s):\nMEASurement<m>:DELay:MARKer"}, {"Level"=2, "Class Only"=TRUE, "Identifier"="", "Descriptive Name"="General Measurements Settings", "Data Type"=0, "Command"="", "Access"=0, "Range Table"="", "Read Callback"="", "Write Callback"="", "Supported Models"="", "Instrument Options"="", "Flags"=0, "Help"="Settings common for all measurements."}, {"Level"=3, "Class Only"=FALSE, "Identifier"="RSRTX_ATTR_MEASUREMENT_ENABLED", "Descriptive Name"="Measurement Enabled", "Data Type"=3, "Command"="MEAS{Measurement}:ENAB", "Access"=2, "Range Table"="", "Read Callback"="", "Write Callback"="", "Supported Models"="", "Instrument Options"="", "Flags"=0, "Help"="Switches the indicated measurement on or off.\n\nAvailable Repeated Capabilities:\nMeasurement: M1, M2, M3, M4, M5, M6, M7, M8\r\n\nRemote-control command(s):\nMEASurement<m>[:ENABle]"}, {"Level"=3, "Class Only"=FALSE, "Identifier"="RSRTX_ATTR_MEASUREMENT_CATEGORY", "Descriptive Name"="Measurement Category", "Data Type"=0, "Command"="MEAS{Measurement}:CAT?", "Access"=0, "Range Table"="rsrtx_rngMeasurementCategory", "Read Callback"="", "Write Callback"="", "Supported Models"="", "Instrument Options"="", "Flags"=0, "Help"="Defines the measurement category.\n\nAvailable Repeated Capabilities:\nMeasurement: M1, M2, M3, M4, M5, M6, M7, M8\r\n\nRemote-control command(s):\nMEASurement<m>:CATegory?"}, {"Level"=3, "Class Only"=FALSE, "Identifier"="RSRTX_ATTR_QUICK_MEASUREMENTS_ENABLE", "Descriptive Name"="Quick Measurements Enable", "Data Type"=4, "Command"="MEAS{Measurement}:AON", "Access"=1, "Range Table"="", "Read Callback"="", "Write Callback"="", "Supported Models"="", "Instrument Options"="", "Flags"=0, "Help"="Enables all additional measurements in all categories of the indicated measurement.\n\nAvailable Repeated Capabilities:\nMeasurement: M1, M2, M3, M4, M5, M6, M7, M8\r\n\nRemote-control command(s):\nMEASurement<m>:AON"}, 
